vi "Circular_Trajectory_planning_of_FCM_with_Time.vi"() -> ()   [LabVIEW 2019]
uses:
  <vilib>/FPGAPlugInAG/sbRIO-9629/niLvFpga_Open_sbRIO-9629.vi
  <vilib>/rvi/interface/common/dynamic/niFpgaDynamicAddResources.vi
  <vilib>/Utility/error.llb/Error Cluster From Error Code.vi
  <vilib>/rvi/errors/niLvFpgaAdjustHostInterfaceError.vi
  <vilib>/FPGAPlugInAG/Dynamic/niLvFpga_Close_Dynamic.vi
  <vilib>/rvi/interface/nirviOpenFPGA/nirviOpenFPGA.xnode
  FPGA Bitfiles/fcmsinglesection_FPGATarget_CloseLoopMotorTu_eGt+d+EV+VE.lvbitx
  Close_Loop_Motor_Tune.vi
  <vilib>/rvi/interface/nirviReadWriteControl/nirviReadWriteControl.xnode
  <vilib>/rvi/interface/nirviCloseFPGA/nirviCloseFPGA.xnode
  NiFpgaLv.dll
  <vilib>/rvi/interface/Simulation/niFpgaSimulationCallBeginRW.vi
panel:
  in  "radius":dbl=0.1
  in  "Degree per Step":dbl=0.0174533
  out "alpha":dbl
  out "L_v":dbl
  out "Tip Position":dbl[](array[numeric])
  in  "Time":dbl
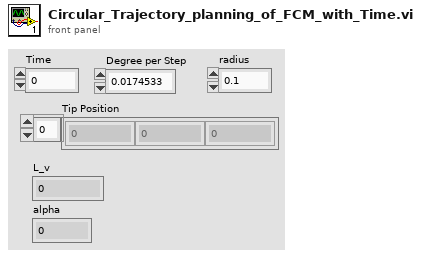
[diagram p1: front panel]
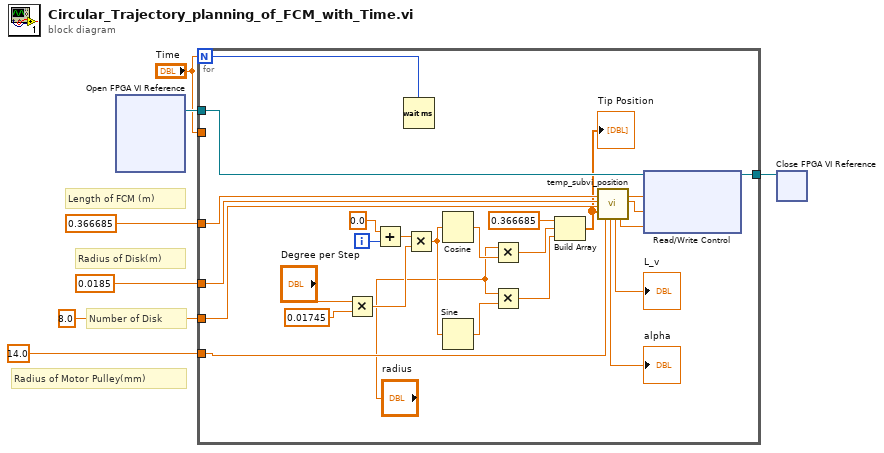
[diagram p0: block diagram]
diagram:
  # "Radius of Motor Pulley(mm)"
  # "Number of Disk"
  # "Radius of Disk(m)"
  # "Length of FCM (m)"
  n1 = xnode "Open FPGA VI Reference"() -> ("FPGA VI Reference Out"=w3:refnum<k20>)  [unwired: 2 in, 1 out]
  n2 = for {
    N: "Time" -> [w9]
    tunnel: 0.366685 ("Length of the FCM (m)") -> [w23]
    tunnel: 0.0185 ("Radius of disk (m)") -> [w22]
    tunnel: 8.0 ("Number of Disks") -> [w21]
    tunnel: 14.0 ("Radius of motor pulley\n (mm)") -> [w20]
    tunnel: w3 -> [w24]
    tunnel: [w15] -> w2
    tunnel: "Time" -> [_]
    i -> [w33]
    n3 = Multiply(x="Degree per Step", y=0.01745) -> (x*y=w11:dbl)
    n4 = Add(x=0.0, y=w33) -> (x+y=w31:dbl)
    n5 = Wait (ms)(milliseconds to wait=w9) -> ()  [unwired: 1 out]
    n6 = Multiply(x=w31, y=w11) -> (x*y=w26:dbl)
    n7 = Cosine(x=w26) -> (cos(x)=w30:dbl)
    n8 = Sine(x=w26) -> (sin(x)=w29:dbl)
    n9 = Multiply(x="radius", y=w30) -> (x*y=w28:dbl)
    n10 = Multiply(x="radius", y=w29) -> (x*y=w27:dbl)
    n11 = Build Array(0.366685, w28, w27) -> (w16:dbl[])
    "Tip Position" <- w16
    n12 = call "temp_subvi_position.vi"("Length of the FCM (m)"=w23, "Radius of disk (m)"=w22, "Number of Disks"=w21, "Tip position"=w16, "Radius of pulley (mm)"=w20) -> ("alpha"=→"alpha":dbl, "L_v"=→"L_v":dbl, "Theta 3"=w17:dbl, "Theta 1"=w19:dbl, "Theta 2"=w18:dbl)  [unwired: 4 in, 6 out]
    n13 = xnode "Read/Write Control"("FPGA VI Reference In"=w24, "desired angle"=w19, "desired angle 2"=w18, "desired angle 3"=w17) -> ("FPGA VI Reference Out"=w15:refnum<k20>)  [unwired: 1 in, 1 out]
  }
  n14 = xnode "Close FPGA VI Reference"("FPGA VI Reference In"=w2) -> ()  [unwired: 1 in, 1 out]
